vi "test init Jl server.vi"(8 "error in (no error)":errorcluster, 11 "Julia user functions script":path=path "C:/_MyOwnDocs/SoftwareDevelopment/Labview2Jl.jl/src/LabVIEW/LV2Julia_examples/jl-scripts/01-add_two_numbers.jl") -> (0 "error out":errorcluster, 2 "Jl Server state out":T1, 3 "timeout?":bool)   [LabVIEW 2018, in "LV-0mq-Julia_roundtrip-lib.lvlib" / "LV2Julia_core.lvlib"]
doc: "Init Julia server & LabView client."
uses:
  LV2Julia_core.lvlib
  Server or client state.ctl
  Commands.ctl
panel:
  out "error out 2":errorcluster
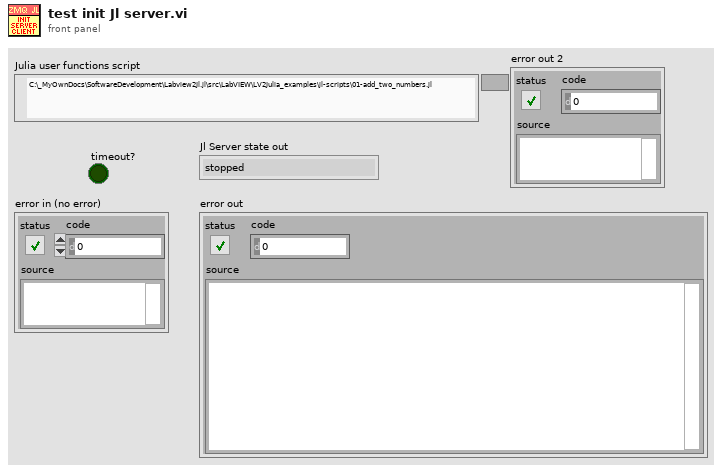
[diagram p1: front panel]
types:
  T1 = typedef "LV-0mq-Julia_roundtrip-lib.lvlib/LV2Julia_core.lvlib/Server or client state.ctl" = enum16{"stopped", "running", "unknown"}
  T2 = typedef "LV-0mq-Julia_roundtrip-lib.lvlib/LV2Julia_core.lvlib/Commands.ctl" = enum16{"Start Jl-server & Init LV-client", "Send request & Get response ", "Stop Jl-server & Cleanup LV-client", "Cleanup LV-client", "Start Jl-server", "Stop Jl-server", "Init LV-Client", "Cleanup LV-Client", "(not allowed)", "Set LV Client state", "Set Jl Server state", "set ZMQ timeout", "read ZMQ timeout", "read-out state"}
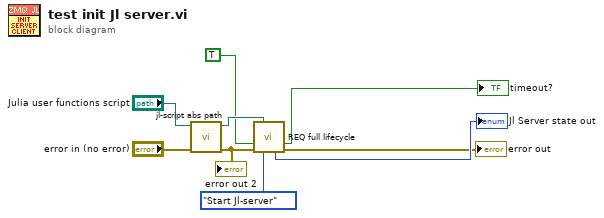
[diagram p0: block diagram]
diagram:
  n1 = call "jl-script abs path.vi"("error in (no error)"="error in (no error)", "Julia user functions script"="Julia user functions script") -> ("error out"=w4:errorcluster, "script abs path"=w3:path)  [unwired: 8 in]
  "error out 2" <- w4
  n2 = call "REQ full lifecycle.vi"("Julia user functions script"=w3, "Force command"=TRUE, "error in"=w4, "command"=Commands."Start Jl-server") -> ("timeout?"=→"timeout?":bool, "Jl Server state out"=→"Jl Server state out":T1, "error out"=→"error out":errorcluster)  [unwired: 5 in, 4 out]
